vi "EHLRequest.vi"(6 "Reply":T1, 9 "Message Data":variant, 11 "Message Queue in":refnum<class "RQMHMessageQueue.lvclass">) -> (0 "error out":errorcluster)   [LabVIEW 2024, in "AddNewEvent.lvlib"]
uses:
  AddNewEvent.lvlib
  JQMHCore/Module/Reply.ctl
  Message Queue_class/RQMHMessageQueue.lvclass
  Message Queue_class/RQMHMessageQueue.lvclass/RQMHMessageQueue.ctl
  Message Queue_class/Delacor_lib_QMH_Enqueue Message (Single).vi
  JQMHCore/Shared/RQMHShared.lvlib
  JQMHCore/Module/RQMHModule.lvclass
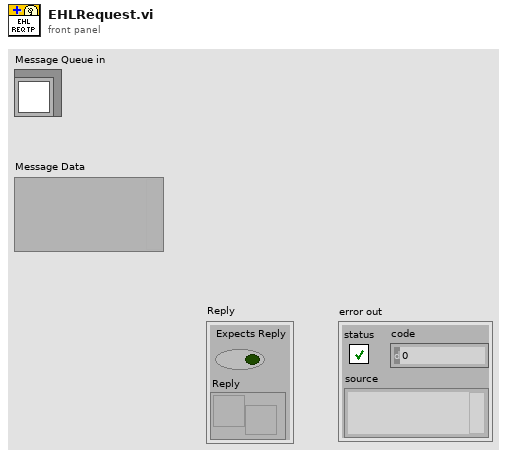
[diagram p1: front panel]
types:
  T1 = typedef "RQMHModule.lvclass/Reply.ctl" = cluster{"Expects Reply":bool, "Reply":refnum<notifier>}
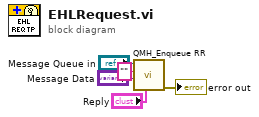
[diagram p0: block diagram]
diagram:
  n1 = call "QMH_Enqueue RR.vi"("Reply"="Reply", "Message Data"="Message Data", "Message"="", "Message Queue in"="Message Queue in") -> ("error out"=→"error out":errorcluster)  [unwired: 6 in, 1 out]
